vi "Send multipart STAT message and wait for reply.vi"(0 "LEIN custom reply Q":T3, 1 "Via master":bool, 2 "Master Address":u8, 5 "LEIN Variation":T4, 7 "Multipart message":T1[](array[typedef]), 11 "error in":errorcluster, 12 "timeout per message":i32) -> (6 "DATA":u8[](array[numeric]), 8 "Data received":bool, 15 "error out":errorcluster)   [LabVIEW 2011]
uses:
  Defenitions/LEIN Structure variations.ctl
  Defenitions/LEIN custom reply Q.ctl
  Defenitions/LEIN Reply Holder.ctl
  Defenitions/LEIN CMD Cluster.ctl
  Defenitions/LEIN CMD List.ctl
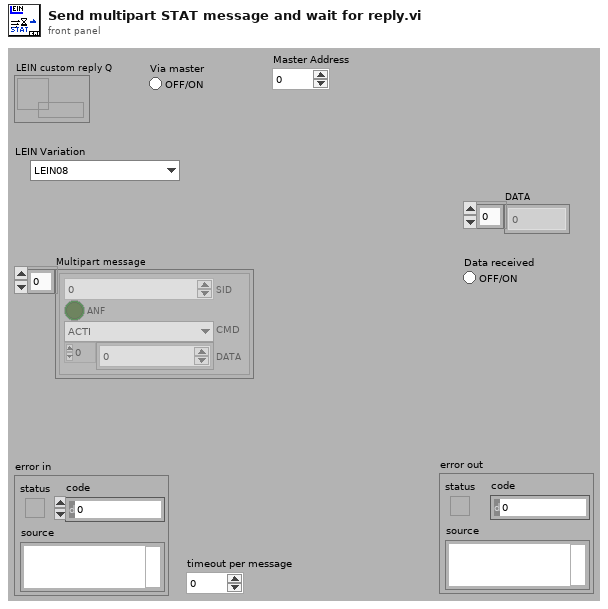
[diagram p1: front panel]
types:
  T1 = typedef "LEIN CMD Cluster.ctl" = cluster{"SID":u8, "ANF":bool, "CMD":T2, "DATA":u8[]}
  T2 = typedef "LEIN CMD List.ctl" = enum8{"ACTI", "TASK", "RES0", "STAT", "RES1", "RES2", "RES3", "USER"}
  T3 = typedef "LEIN custom reply Q.ctl" = refnum<queue>
  T4 = typedef "LEIN Structure variations.ctl" = enum16{"LEIN08", "LEIN31", "LEIN63"}
  T5 = typedef "LEIN Reply Holder.ctl" = cluster{"Reply msg(cmdif no reply)":T1, "Reply time":timestamp, "Valid reply":bool}
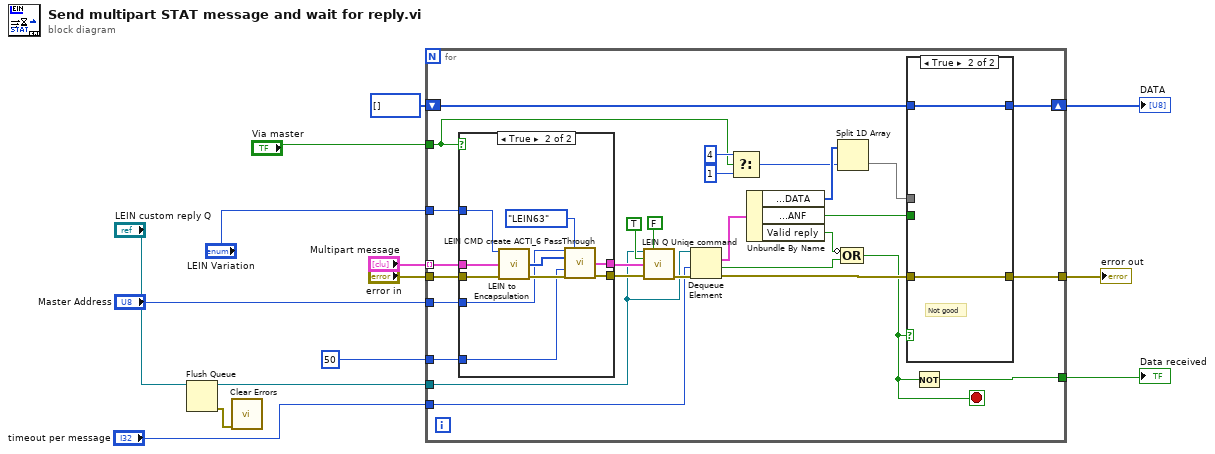
[diagram p0: block diagram]
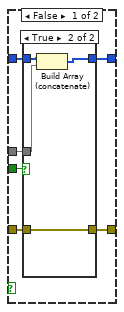
[diagram p2: hidden frame]
diagram:
  n1 = Flush Queue(queue="LEIN custom reply Q") -> (queue out=w2:T3, error out=w1:errorcluster)  [unwired: 1 in, 1 out]
  n2 = call <vilib>:"Clear Errors.vi"("error in (no error)"=w1) -> ()  [unwired: 6 in, 1 out]
  n3 = for {
    tunnel: [w29] -> w10
    tunnel: "error in" -> [w40]
    tunnel: "Multipart message" -> [w35] mode=indexing
    tunnel: w2 -> [w32]
    tunnel: "Via master" -> [w15]
    tunnel: "LEIN Variation" -> [w38]
    tunnel: "Master Address" -> [w37]
    tunnel: u16 50 ("ACTI 6 timeout") -> [w36]
    tunnel: [w31] -> w14
    shift-right: [w22] -> w13
    shift-left: u8[] [] ("DATA") -> [w21]
    tunnel: "timeout per message" -> [w20]
    stop <- w26 stop-if-true
    n4 = case shown="True" w15 {
      tunnel: [w57 w65] -> w34
      tunnel: [w58 w64] -> w39
      tunnel: w40 -> [w58 w63]
      tunnel: w35 -> [w57 w62]
      tunnel: w37 -> [_ w61]
      tunnel: w36 -> [_ w60]
      tunnel: w38 -> [_ w59]
      frame False {
      }
      frame True {
        n5 = call "LEIN to Encapsulation.vi"("LEIN Variation"=w59, "CMD"=w62, "error in (no error)"=w63) -> ("Data and header"=w66:u8[], "error out"=w67:errorcluster)  [unwired: 8 in, 3 out]
        n6 = call "LEIN CMD create ACTI_6 PassThrough.vi"("SID"=w61, "LEIN Variation"=LEIN_Structure_variations."LEIN63", "LEIN ecapsulated data (header and data)"=w66, "Sub Timeout (ms)"=w60, "error in (no error)"=w67) -> ("CMD"=w65:T1, "error out"=w64:errorcluster)  [unwired: 9 in]
      }
    }
    n7 = call "LEIN Q Uniqe command.vi"("LEIN custom reply Q"=w32, "Retry on err (F)"=FALSE, "Custom Q(F)"=TRUE, "CMD"=w34, "error in"=w39) -> ("error out"=w33:errorcluster)  [unwired: 10 in]
    n8 = Dequeue Element(queue=w32, timeout in ms (-1)=w20, error in (no error)=w33) -> (element=w25:T5, timed out?=w28:bool, error out=w30:errorcluster)  [unwired: 1 out]
    n9 = Select(t=4 ("index"), s=w15, f=1 ("index")) -> (s? t:f=w17:i32)
    n10 = Unbundle By Name(w25) -> ("Reply msg(cmdif no reply).DATA"=w23:u8[], "Reply msg(cmdif no reply).ANF"=w24:bool, "Valid reply"=w27:bool)
    n11 = Split 1D Array(array=w23, index=w17) -> (second subarray=w19:u8[])  [unwired: 1 out]
    n12 = Compound Arithmetic op=OR(invert w27, w28) -> (w26:bool)
    n13 = case shown="True" w26 {
      tunnel: w30 -> [w48 w56]
      tunnel: [w43 w56] -> w29
      tunnel: w24 -> [w47 _]
      tunnel: w19 -> [w46 _]
      tunnel: [w45 w55] -> w22
      tunnel: w21 -> [w44 w55]
      frame False {
        n14 = case shown="True" w47 {
          tunnel: w48 -> [w49 w51]
          tunnel: w46 -> [_ w53]
          tunnel: [w50 w52] -> w45
          tunnel: w44 -> [w50 w54]
          tunnel: [w49 w51] -> w43
          frame False {
          }
          frame True {
            n15 = Build Array (concatenate)(w54, w53) -> (w52:u8[])
          }
        }
      }
      frame True {
        # "Not good"
      }
    }
    n16 = Not(x=w26) -> (.not. x?=w31:bool)
  }
  "Data received" <- w14
  "DATA" <- w13
  "error out" <- w10
